vi "Load nsp File.vi"(8 "error in":errorcluster, 11 "file path (use dialog)":path) -> (0 "error out":errorcluster, 1 "df (Hz)":sgl, 2 "Sample points":i32, 3 "Spectrum data":sgl[][](array[numeric]), 4 "Infos":string[][](table), 5 "Spectrum of":string)   [LabVIEW 2019, in "Nanonis Prog Interface.lvlib"]
uses:
  <userlib>/Nanonis Prog Interface V5/Nanonis Prog Interface.lvlib
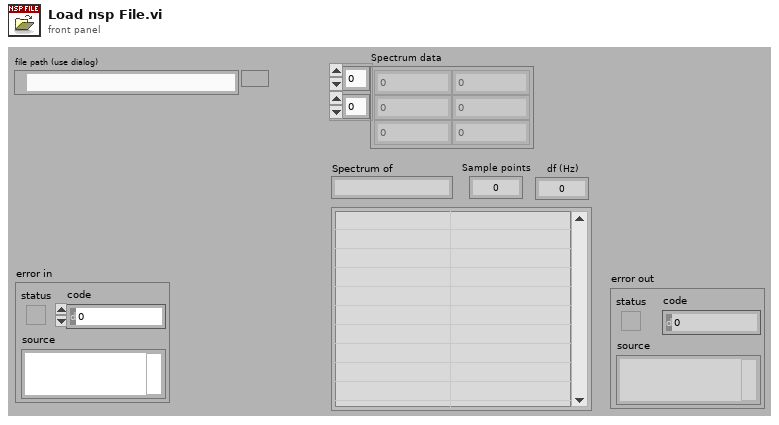
[diagram p1: front panel]
types:
  T1 = enum16{"big-endian, network order", "native, host order", "little-endian"}
  T2 = cluster{"Signal":string, "df":sgl, "starttime":timestamp, "endtime":timestamp, "# lines":i32, "# points":i32, "file":path, "Parameters":string[][], "Number of rows":i32, "Number of cols":i32}
  T3 = typedef "LVDateTimeRec.ctl" = cluster{"fractional second":dbl, "second":i32, "minute":i32, "hour":i32, "day of month":i32, "month":i32, "year":i32, "day of week":i32, "day of year":i32, "DST":i32}
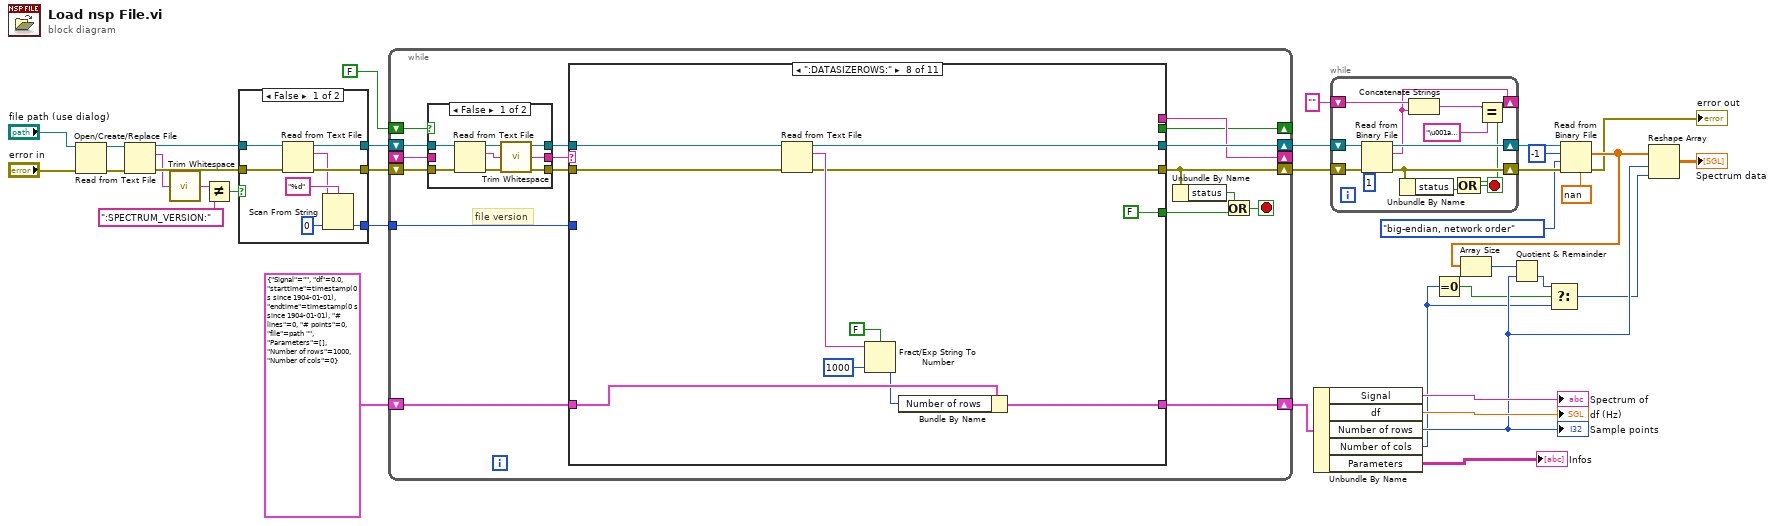
[diagram p0: block diagram]
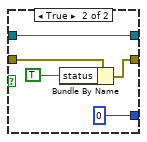
[diagram p2: hidden frame]
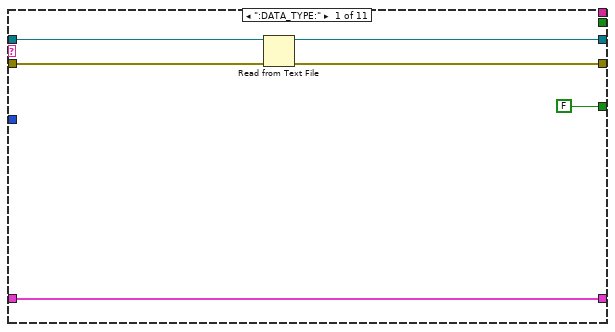
[diagram p4: hidden frame]
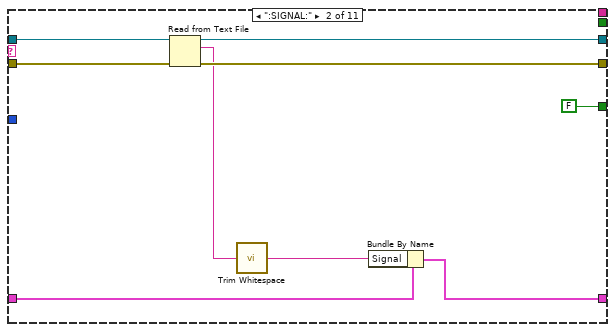
[diagram p5: hidden frame]
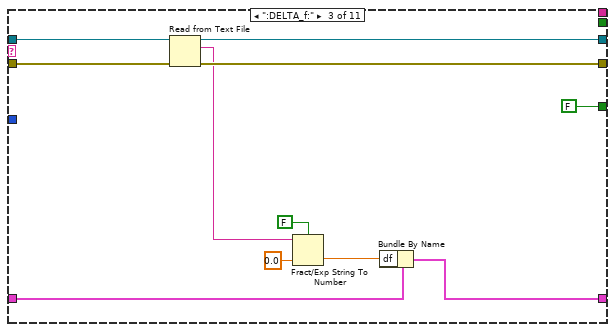
[diagram p6: hidden frame]
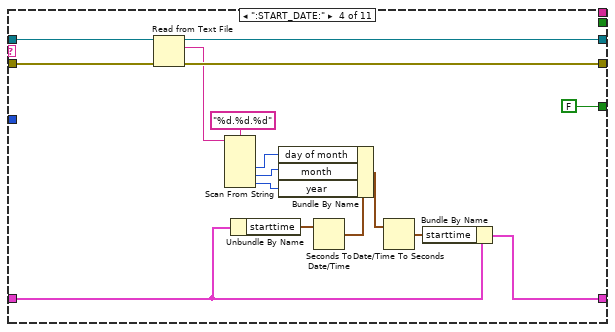
[diagram p7: hidden frame]
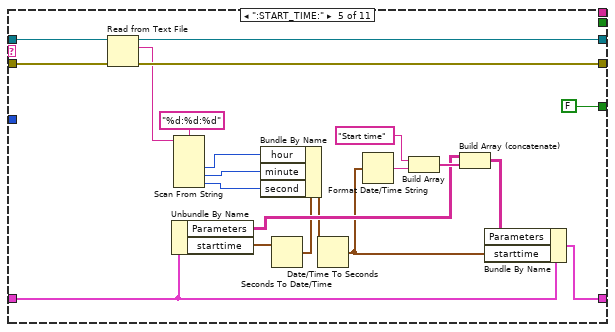
[diagram p8: hidden frame]
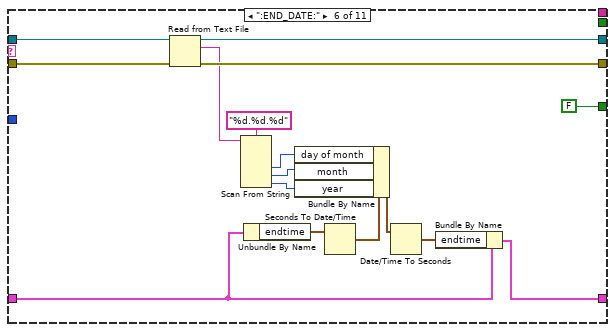
[diagram p9: hidden frame]
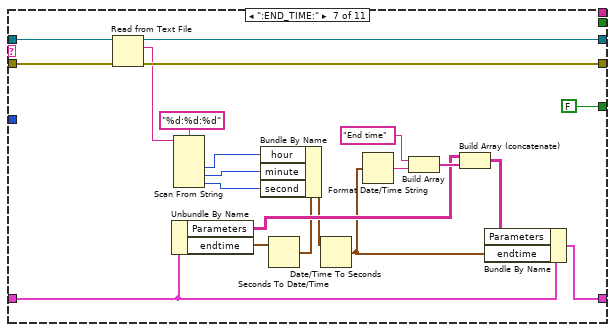
[diagram p10: hidden frame]
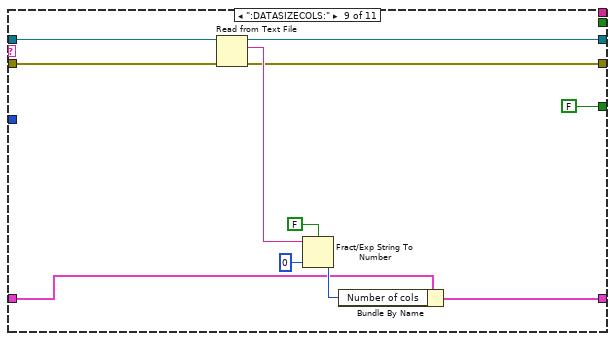
[diagram p11: hidden frame]
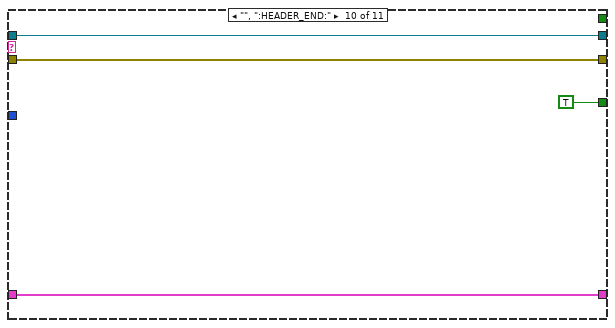
[diagram p12: hidden frame]
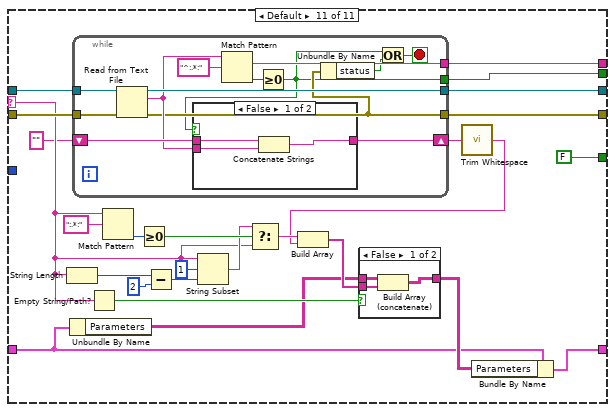
[diagram p13: hidden frame]
diagram:
  n1 = Open/Create/Replace File(file path (use dialog)="file path (use dialog)", error in="error in") -> (refnum out=w33:refnum<file>, error out=w32:errorcluster)  [unwired: 4 in, 1 out]
  n2 = Read from Text File(file (use dialog)=w33, error in=w32) -> (refnum out=w28:refnum<file>, text=w13:string, error out=w31:errorcluster)  [unwired: 2 in, 1 out]
  n3 = call <vilib>:"Trim Whitespace.vi"("string"=w13) -> ("trimmed string"=w29:string)  [unwired: 1 in]
  n4 = Not Equal?(x=w29, y=":SPECTRUM_VERSION:") -> (x != y?=w34:bool)
  n5 = case shown="False" w34 {
    tunnel: w31 -> [w37 w49]
    tunnel: [w44 w48] -> w30
    tunnel: w28 -> [w38 w46]
    tunnel: [w43 w46] -> w27
    tunnel: [w40 0 ("default value 1")] -> w26
    frame False {
      n6 = Read from Text File(file (use dialog)=w38, error in=w37) -> (refnum out=w43:refnum<file>, text=w41:string, error out=w44:errorcluster)  [unwired: 2 in, 1 out]
      n7 = Scan From String(format string="%d", input string=w41, default 1=0 ("default value 1")) -> (output 1=w40:i32)  [unwired: 2 in, 3 out]
    }
    frame True {
      n8 = Bundle By Name(cluster=w49, "status"=TRUE) -> (w48:errorcluster)
    }
  }
  n9 = while {
    shift-right: [w65] -> w18
    shift-left: T2 {"Signal"="", "df"=0.0, "starttime"=timestamp(0 s since 1904-01-01), "endtime"=timestamp(0 s since 1904-01-01), "# lines"=0, "# points"=0, "file"=path "", "Parameters"=[], "Number of rows"=1000, "Number of cols"=0} ("Scan-Databuffer-attributes") -> [w66]
    shift-right: [w61] -> w22
    shift-left: w30 -> [w60]
    shift-right: [w55] -> w23
    shift-left: w27 -> [w58]
    tunnel: w26 -> [w54]
    shift-right: [w50] -> _
    shift-left: FALSE -> [w53]
    shift-right: [w51] -> _
    shift-left: _ -> [w52]
    stop <- w62 stop-if-true
    # "file version"
    n10 = case shown="False" w53 {
      tunnel: w60 -> [w67 w74]
      tunnel: [w71 w74] -> w59
      tunnel: w58 -> [w68 w73]
      tunnel: [w70 w73] -> w57
      tunnel: [w69 w75] -> w56
      tunnel: w52 -> [_ w75]
      frame False {
        n11 = Read from Text File(file (use dialog)=w68, error in=w67) -> (refnum out=w70:refnum<file>, text=w72:string, error out=w71:errorcluster)  [unwired: 2 in, 1 out]
        n12 = call <vilib>:"Trim Whitespace.vi"("string"=w72) -> ("trimmed string"=w69:string)  [unwired: 1 in]
      }
      frame True {
      }
    }
    n13 = case shown="\":DATASIZEROWS:\"" w56 {
      selector: w56 -> [_ _ _ _ _ _ _ _ _ _ w208]
      tunnel: w57 -> [w77 w83 w92 w103 w119 w140 w156 w177 w188 w199 w202]
      tunnel: [FALSE ("true") FALSE ("true") FALSE ("true") FALSE ("true") FALSE ("true") FALSE ("true") FALSE ("true") FALSE ("true") FALSE ("true") TRUE ("true") FALSE ("true")] -> w63
      tunnel: w66 -> [w79 w87 w98 w106 w129 w145 w166 w181 w192 w200 w219]
      tunnel: [w79 w86 w97 w107 w138 w146 w175 w178 w191 w200 w221] -> w65
      tunnel: [w80 w89 w100 w116 w132 w153 w169 w182 w190 w199 w225] -> w55
      tunnel: w59 -> [w76 w82 w91 w102 w118 w139 w155 w176 w187 w198 w226]
      tunnel: [w81 w88 w99 w109 w131 w148 w168 w183 w189 w198 w224] -> w61
      tunnel: w54 -> [_ _ _ _ _ _ _ _ _ _ _]
      tunnel: [_ _ _ _ _ _ _ _ _ _ w207] -> w51
      tunnel: [_ _ _ _ _ _ _ _ _ _ w206] -> w50
      frame ":DATA_TYPE:" {
        n14 = Read from Text File(file (use dialog)=w77, error in=w76) -> (refnum out=w80:refnum<file>, error out=w81:errorcluster)  [unwired: 2 in, 2 out]
      }
      frame ":SIGNAL:" {
        n15 = Read from Text File(file (use dialog)=w83, error in=w82) -> (refnum out=w89:refnum<file>, text=w85:string, error out=w88:errorcluster)  [unwired: 2 in, 1 out]
        n16 = call <vilib>:"Trim Whitespace.vi"("string"=w85) -> ("trimmed string"=w84:string)  [unwired: 1 in]
        n17 = Bundle By Name(cluster=w87, "Signal"=w84) -> (w86:T2)
      }
      frame ":DELTA_f:" {
        n18 = Read from Text File(file (use dialog)=w92, error in=w91) -> (refnum out=w100:refnum<file>, text=w96:string, error out=w99:errorcluster)  [unwired: 2 in, 1 out]
        n19 = Fract/Exp String To Number(use system decimal point (T)=FALSE, string=w96, default (0 dbl)=sgl 0.0 ("default (0 DBL)")) -> (number=w95:sgl)  [unwired: 1 in, 1 out]
        n20 = Bundle By Name(cluster=w98, "df"=w95) -> (w97:T2)
      }
      frame ":START_DATE:" {
        n21 = Read from Text File(file (use dialog)=w103, error in=w102) -> (refnum out=w116:refnum<file>, text=w108:string, error out=w109:errorcluster)  [unwired: 2 in, 1 out]
        n22 = Scan From String(format string="%d.%d.%d", input string=w108) -> (output 1=w112:i32, output 2=w111:i32, output 3=w110:i32)  [unwired: 5 in, 3 out]
        n23 = Unbundle By Name(w106) -> ("starttime"=w105:timestamp)
        n24 = Seconds To Date/Time(time stamp (now)=w105) -> (date time rec=w115:T3)  [unwired: 1 in]
        n25 = Bundle By Name(cluster=w115, "day of month"=w112, "month"=w111, "year"=w110) -> (w104:T3)
        n26 = Date/Time To Seconds(2:w104) -> (0:w114:timestamp)  [unwired: 1 in]
        n27 = Bundle By Name(cluster=w106, "starttime"=w114) -> (w107:T2)
      }
      frame ":START_TIME:" {
        n28 = Read from Text File(file (use dialog)=w119, error in=w118) -> (refnum out=w132:refnum<file>, text=w130:string, error out=w131:errorcluster)  [unwired: 2 in, 1 out]
        n29 = Unbundle By Name(w129) -> ("Parameters"=w125:string[][], "starttime"=w123:timestamp)
        n30 = Scan From String(format string="%d:%d:%d", input string=w130) -> (output 1=w136:i32, output 2=w135:i32, output 3=w134:i32)  [unwired: 5 in, 3 out]
        n31 = Seconds To Date/Time(time stamp (now)=w123) -> (date time rec=w122:T3)  [unwired: 1 in]
        n32 = Bundle By Name(cluster=w122, "hour"=w136, "minute"=w135, "second"=w134) -> (w121:T3)
        n33 = Date/Time To Seconds(2:w121) -> (0:w120:timestamp)  [unwired: 1 in]
        n34 = Format Date/Time String(seconds (now)=w120) -> (date/time string=w127:string)  [unwired: 2 in]
        n35 = Build Array("Start time" ("format string"), w127) -> (w126:string[])
        n36 = Build Array (concatenate)(w125, w126) -> (w124:string[][])
        n37 = Bundle By Name(cluster=w129, "Parameters"=w124, "starttime"=w120) -> (w138:T2)
      }
      frame ":END_DATE:" {
        n38 = Read from Text File(file (use dialog)=w140, error in=w139) -> (refnum out=w153:refnum<file>, text=w147:string, error out=w148:errorcluster)  [unwired: 2 in, 1 out]
        n39 = Scan From String(format string="%d.%d.%d", input string=w147) -> (output 1=w151:i32, output 2=w150:i32, output 3=w149:i32)  [unwired: 5 in, 3 out]
        n40 = Unbundle By Name(w145) -> ("endtime"=w143:timestamp)
        n41 = Seconds To Date/Time(time stamp (now)=w143) -> (date time rec=w144:T3)  [unwired: 1 in]
        n42 = Bundle By Name(cluster=w144, "day of month"=w151, "month"=w150, "year"=w149) -> (w142:T3)
        n43 = Date/Time To Seconds(2:w142) -> (0:w141:timestamp)  [unwired: 1 in]
        n44 = Bundle By Name(cluster=w145, "endtime"=w141) -> (w146:T2)
      }
      frame ":END_TIME:" {
        n45 = Read from Text File(file (use dialog)=w156, error in=w155) -> (refnum out=w169:refnum<file>, text=w167:string, error out=w168:errorcluster)  [unwired: 2 in, 1 out]
        n46 = Unbundle By Name(w166) -> ("Parameters"=w162:string[][], "endtime"=w160:timestamp)
        n47 = Scan From String(format string="%d:%d:%d", input string=w167) -> (output 1=w173:i32, output 2=w172:i32, output 3=w171:i32)  [unwired: 5 in, 3 out]
        n48 = Seconds To Date/Time(time stamp (now)=w160) -> (date time rec=w159:T3)  [unwired: 1 in]
        n49 = Bundle By Name(cluster=w159, "hour"=w173, "minute"=w172, "second"=w171) -> (w158:T3)
        n50 = Date/Time To Seconds(2:w158) -> (0:w157:timestamp)  [unwired: 1 in]
        n51 = Format Date/Time String(seconds (now)=w157) -> (date/time string=w164:string)  [unwired: 2 in]
        n52 = Build Array("End time" ("format string"), w164) -> (w163:string[])
        n53 = Build Array (concatenate)(w162, w163) -> (w161:string[][])
        n54 = Bundle By Name(cluster=w166, "Parameters"=w161, "endtime"=w157) -> (w175:T2)
      }
      frame ":DATASIZEROWS:" {
        n55 = Read from Text File(file (use dialog)=w177, error in=w176) -> (refnum out=w182:refnum<file>, text=w186:string, error out=w183:errorcluster)  [unwired: 2 in, 1 out]
        n56 = Fract/Exp String To Number(use system decimal point (T)=FALSE, string=w186, default (0 dbl)=1000 ("default (0 DBL)")) -> (number=w179:i32)  [unwired: 1 in, 1 out]
        n57 = Bundle By Name(cluster=w181, "Number of rows"=w179) -> (w178:T2)
      }
      frame ":DATASIZECOLS:" {
        n58 = Read from Text File(file (use dialog)=w188, error in=w187) -> (refnum out=w190:refnum<file>, text=w197:string, error out=w189:errorcluster)  [unwired: 2 in, 1 out]
        n59 = Fract/Exp String To Number(use system decimal point (T)=FALSE, string=w197, default (0 dbl)=0 ("default (0 DBL)")) -> (number=w194:i32)  [unwired: 1 in, 1 out]
        n60 = Bundle By Name(cluster=w192, "Number of cols"=w194) -> (w191:T2)
      }
      frame "", ":HEADER_END:" {
      }
      frame Default {
        n61 = String Length(string=w208) -> (length=w215:i32)
        n62 = Unbundle By Name(w219) -> ("Parameters"=w218:string[][])
        n63 = while {
          tunnel: w202 -> [w229]
          tunnel: w226 -> [w228]
          tunnel: [w240] -> w225
          tunnel: [w233] -> w224
          tunnel: [w237] -> w207
          tunnel: [w231] -> w206
          shift-right: [w235] -> w204
          shift-left: "" ("regular expression") -> [w236]
          stop <- w230 stop-if-true
          n64 = Read from Text File(file (use dialog)=w229, error in=w228) -> (refnum out=w240:refnum<file>, text=w234:string, error out=w233:errorcluster)  [unwired: 2 in, 1 out]
          n65 = Match Pattern(string=w234, regular expression="^:.*:") -> (match substring=w237:string, offset past match=w239:i32)  [unwired: 1 in, 2 out]
          n66 = Greater Or Equal To 0?(x=w239) -> (x >= 0?=w231:bool)
          n67 = case shown="False" w231 {
            tunnel: w236 -> [w243 w244]
            tunnel: [w242 w244] -> w235
            tunnel: w234 -> [w241 _]
            frame False {
              n68 = Concatenate Strings(w243, w241) -> (w242:string)
            }
            frame True {
            }
          }
          n69 = Unbundle By Name(w233) -> ("status"=w232:bool)
          n70 = Or(x=w231, y=w232) -> (x .or. y?=w230:bool)
        }
        n71 = Empty String/Path?(string/path=w208) -> (empty?=w222:bool)
        n72 = Match Pattern(string=w208, regular expression=":.*:") -> (offset past match=w212:i32)  [unwired: 1 in, 3 out]
        n73 = Greater Or Equal To 0?(x=w212) -> (x >= 0?=w211:bool)
        n74 = Subtract(x=w215, y=2) -> (x-y=w213:i32)
        n75 = String Subset(string=w208, offset (0)=1, length (rest)=w213) -> (substring=w210:string)
        n76 = Select(t=w210, s=w211, f=w208) -> (s? t:f=w209:string)
        n77 = call <vilib>:"Trim Whitespace.vi"("string"=w204) -> ("trimmed string"=w203:string)  [unwired: 1 in]
        n78 = Build Array(w209, w203) -> (w223:string[])
        n79 = case shown="False" w222 {
          tunnel: w218 -> [w247 w248]
          tunnel: w223 -> [w246 _]
          tunnel: [w245 w248] -> w220
          frame False {
            n80 = Build Array (concatenate)(w247, w246) -> (w245:string[][])
          }
          frame True {
          }
        }
        n81 = Bundle By Name(cluster=w219, "Parameters"=w220) -> (w221:T2)
      }
    }
    n82 = Unbundle By Name(w61) -> ("status"=w64:bool)
    n83 = Or(x=w64, y=w63) -> (x .or. y?=w62:bool)
  }
  n84 = Unbundle By Name(w18) -> ("Signal"=→"Spectrum of":string, "df"=→"df (Hz)":sgl, "Number of rows"=w9:i32, "Number of cols"=w6:i32, "Parameters"=→"Infos":string[][])
  "Sample points" <- w9
  n85 = while {
    shift-right: [w251] -> _
    shift-left: "" -> [w260]
    shift-right: [w257] -> w20
    shift-left: w22 -> [w249]
    shift-right: [w259] -> w21
    shift-left: w23 -> [w250]
    stop <- w254 stop-if-true
    n86 = Read from Binary File(8:w249, 10:1 ("count"), 11:w250) -> (0:w257:errorcluster, 2:w251:string, 3:w259:refnum<file>)  [unwired: 3 in, 1 out]
    n87 = Unbundle By Name(w257) -> ("status"=w256:bool)
    n88 = Concatenate Strings(w260, w251) -> (w252:string)
    n89 = Equal?(x=w252, y="\u001a\u0004") -> (x = y?=w255:bool)
    n90 = Compound Arithmetic op=OR(w255, w256) -> (w254:bool)
  }
  n91 = Equal To 0?(x=w6) -> (x = 0?=w8:bool)
  n92 = Read from Binary File(5:sgl nan ("element"), 8:w20, 9:T1."big-endian, network order" ("byte order (0:big-endian, network order)"), 10:-1 ("count (1)"), 11:w21) -> (0:→"error out":errorcluster, 2:w11:sgl[])  [unwired: 1 in, 2 out]
  n93 = Array Size(array=w11) -> (size(s)=w10:i32)
  n94 = Quotient & Remainder(x=w10, y=w9) -> (floor(x/y)=w7:i32)  [unwired: 1 out]
  n95 = Select(t=w7, s=w8, f=w6) -> (s? t:f=w5:i32)
  n96 = Reshape Array(w11, w9, w5) -> (→"Spectrum data":sgl[][])
